vi "worksheet print area.vi"(6 "last_col":u16, 7 "last_row":u32, 8 "error in (no error)":errorcluster, 9 "first_col":u16, 10 "first_row":u32, 11 "worksheet":u32) -> (0 "error out":errorcluster, 3 "function return":u32(ring))   [LabVIEW 2015, in "xlsxwriter.lvlib"]
doc: "lxw_error worksheet_print_area(lxw_worksheet worksheet, lxw_row_t first_row, lxw_col_t first_col, lxw_row_t last_row, lxw_col_t last_col);"
uses:
  xlsxwriter.lvlib
  xlsxwriter.dll
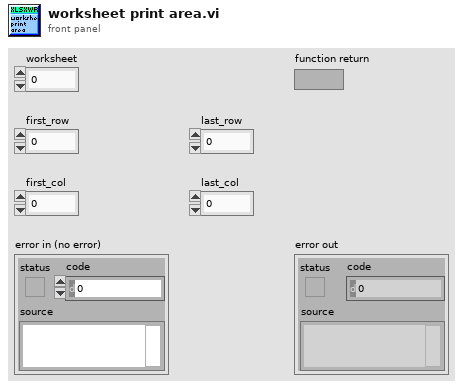
[diagram p1: front panel]
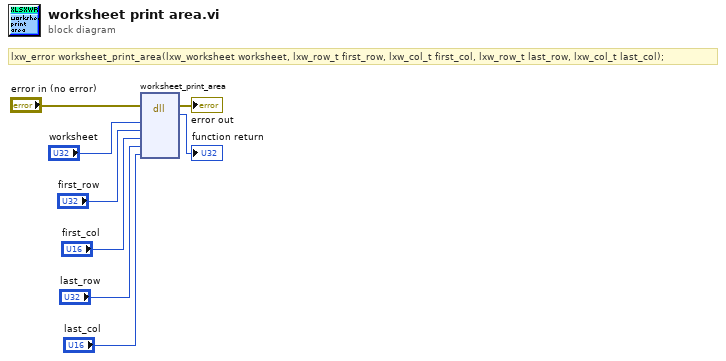
[diagram p0: block diagram]
diagram:
  # "lxw_error worksheet_print_area(lxw_worksheet worksheet, lxw_row_t first_row, lxw_col_t first_col, lxw_row_t last_row, lxw_col_t last_col);"
  n1 = dll-call lib="C:/Users/WDAGUtilityAccount/Desktop/lv_vis_added_cell/xlsxwriter.*" fn="worksheet_print_area"(error in="error in (no error)", "worksheet"="worksheet", "first_row"="first_row", "first_col"="first_col", "last_row"="last_row", "last_col"="last_col") -> (error out=→"error out":errorcluster, →"function return":u32)  [unwired: 7 in, 1 out]
